vi "Select Measurement Listbox.vi"(6 "Cluster in":T3, 8 "error in (no error)":errorcluster, 9 "ThresholdLimits":refnum<vi>, 10 "Coords":T4, 11 "References in":T1) -> (0 "error out":errorcluster, 1 "Enable Disable button state":bool, 2 "Tick Marked?":bool, 3 "Cluster out":T3)   [LabVIEW 2019, in "ZenGage v3.0 UI.lvclass"]
doc: "This VI identifies selection of measurement in list and displays corresponding Lower Limit, Upper Limit, Lower Control Limit and Upper Control Limit values."
uses:
  ZenGage v3.0 UI.lvclass
  <vilib>/Utility/miscctls.llb/LVPositionTypeDef.ctl
  <vilib>/Utility/miscctls.llb/LVPoint32TypeDef.ctl
panel:
  out "References in":T1
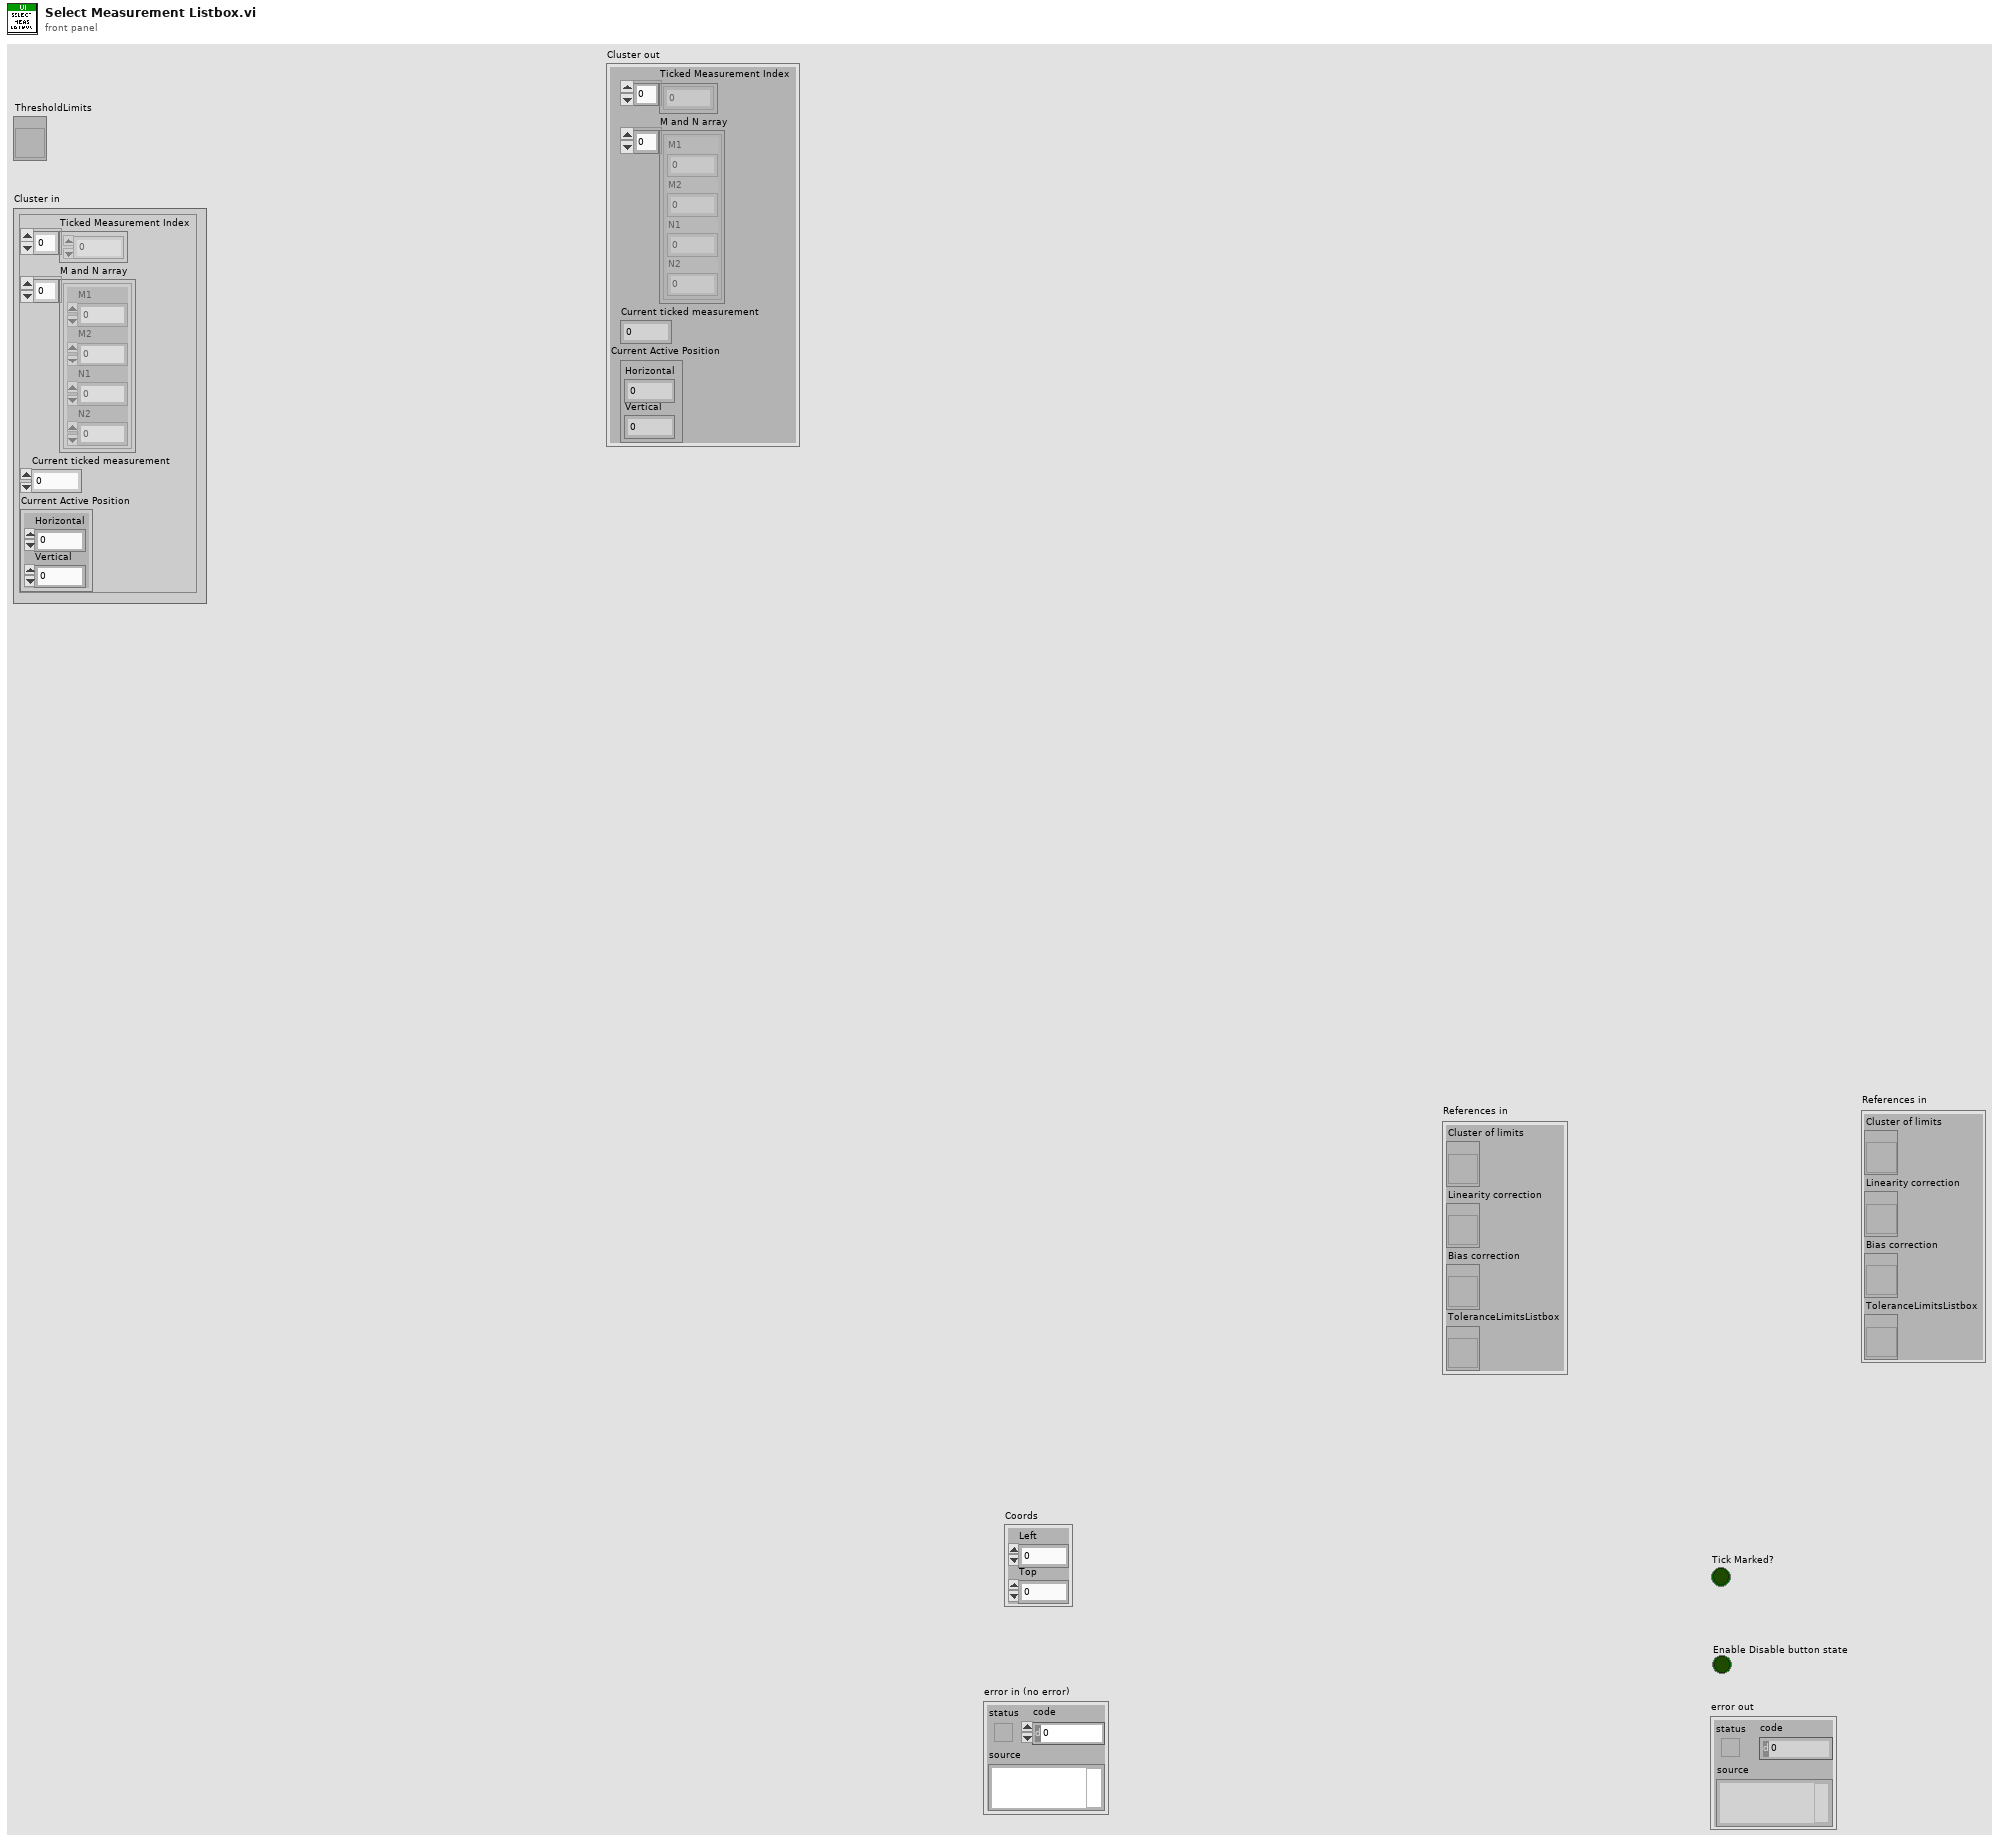
[diagram p1: front panel]
types:
  T1 = cluster{"Cluster of limits":refnum<vi>, "Linearity correction":refnum<vi>, "Bias correction":refnum<vi>, "ToleranceLimitsListbox":refnum<vi>}
  T2 = typedef "LVPoint32TypeDef.ctl" = cluster{"Horizontal":i32, "Vertical":i32}
  T3 = cluster{"Ticked Measurement Index":u32[], "M and N array":cluster{"M1":u64, "M2":u64, "N1":u64, "N2":u64}[], "Current ticked measurement":dbl, "Current Active Position":T2}
  T4 = typedef "LVPositionTypeDef.ctl" = cluster{"Left":i32, "Top":i32}
  T5 = cluster{"Lower Limit":dbl, "Upper Limit":dbl, "Lower Control Limit":dbl, "Upper Control Limit":dbl}
  T6 = enum8{"Enabled", "Disabled", "Disabled and Grayed Out"}
  T7 = cluster{"M1":u64, "M2":u64, "N1":u64, "N2":u64}[]
  T8 = typedef "LVRowAndColumnTypeDef.ctl" = cluster{"Row":i32, "Column":i32}
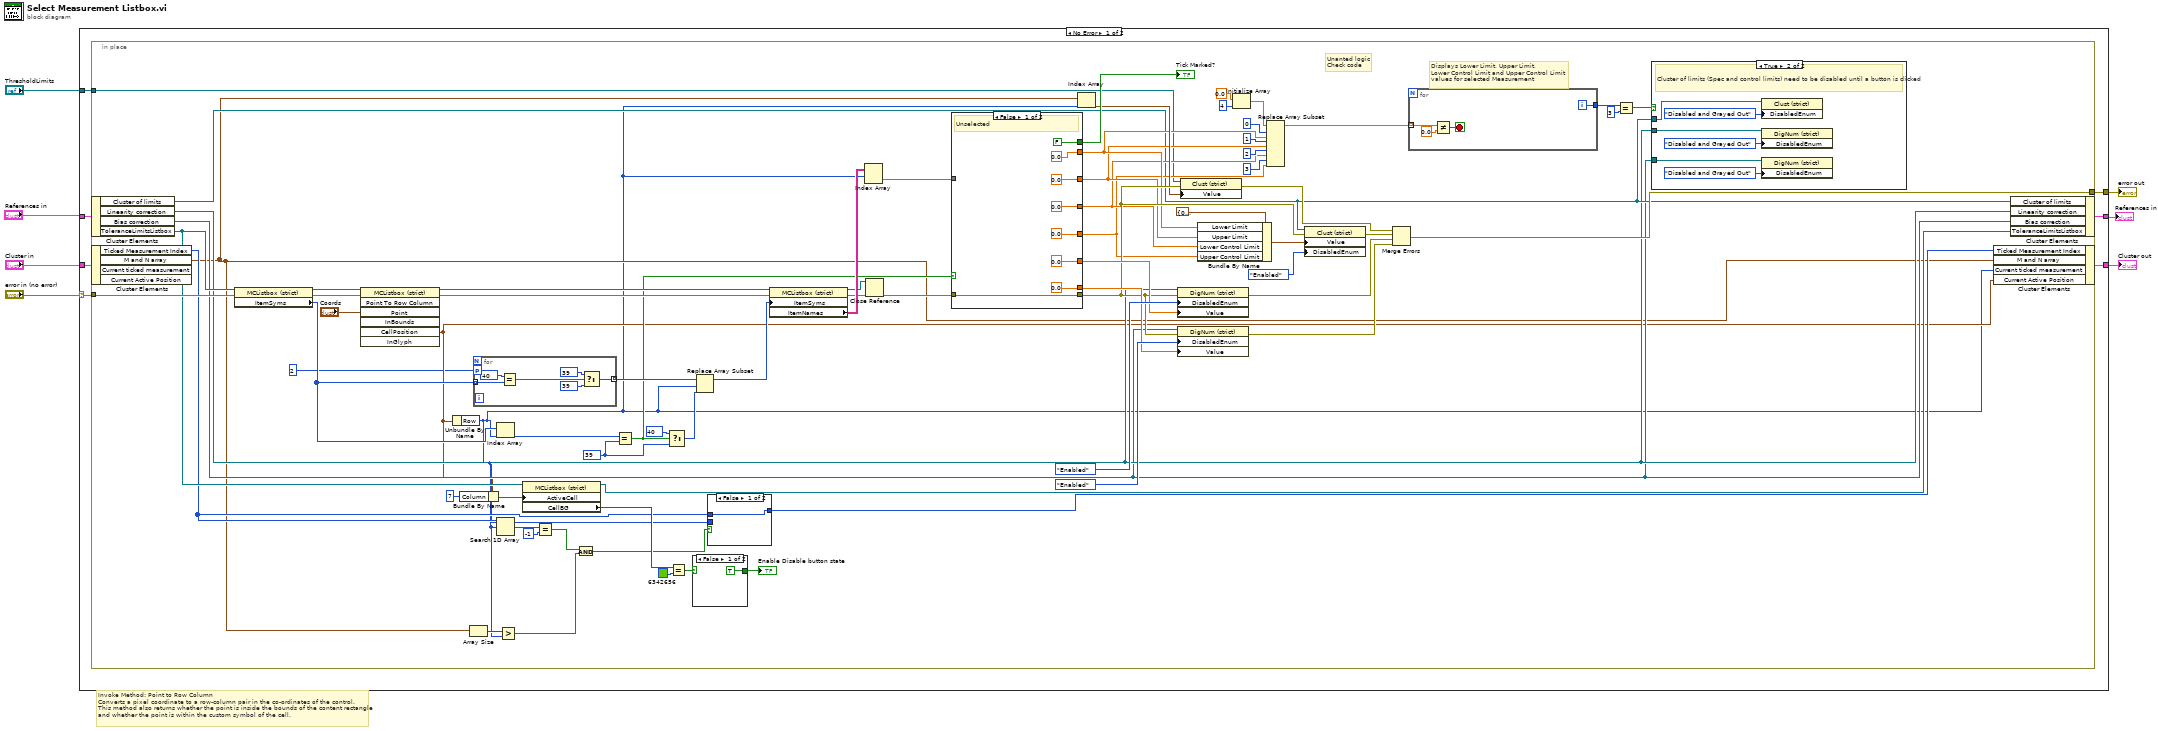
[diagram p0: block diagram]
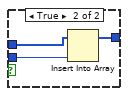
[diagram p2: hidden frame]
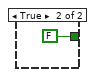
[diagram p3: hidden frame]
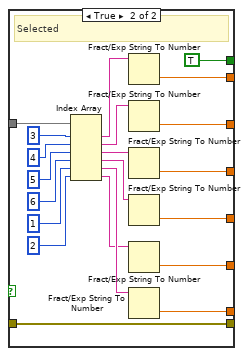
[diagram p5: hidden frame]
diagram:
  # "Invoke Method: Point to Row Column\nConverts a pixel coordinate to a row-column pair in the co-ordinates of the control.\nThis method also returns whether the point is inside the bounds of the content rectangle\nand whether the point is within the custom symbol of the cell."
  n1 = case shown="No Error" "error in (no error)" {
    selector: "error in (no error)" -> [w14 w141]
    tunnel: [w13 w141] -> w6
    tunnel: [w11 w140] -> w1
    tunnel: "References in" -> [w12 w140]
    tunnel: "ThresholdLimits" -> [w10 _]
    tunnel: "Cluster in" -> [w9 w139]
    tunnel: [w8 w139] -> w3
    frame No Error {
      n2 = in-place {
        in-place-border: w14 -> [w49]
        in-place-border: [w47] -> w13
        in-place-border: w10 -> [w25]
        w77 = 39
        # "Unanted logic\nCheck code"
        # "Displays Lower Limit, Upper Limit,\nLower Control Limit and Upper Control Limit\nvalues for selected Measurement"
        n3 = in-place-cluster #1(w12) -> ("Cluster of limits"=w29:refnum<vi>, "Linearity correction"=w28:refnum<vi>, "Bias correction"=w27:refnum<vi>, "ToleranceLimitsListbox"=w30:refnum<vi>)
        n4 = in-place-cluster #2(w9) -> ("Ticked Measurement Index"=w24:u32[], "M and N array"=w18:T7)  [unwired: 2 out]
        n5 = property on="Property Node" class="MCListbox (strict)"(reference=w30, error in=w49) -> (reference out=w85:refnum<vi>, error out=w86:errorcluster, "ItemSyms"=w75:i32[])
        n6 = invoke on="Invoke Node" class="MCListbox (strict)" method="Point To Row Column"(reference=w85, error in=w86, "Point"="Coords") -> (reference out=w84:refnum<vi>, error out=w83:errorcluster, "CellPosition"=w22:T8)  [unwired: 4 in, 4 out]
        n7 = Unbundle By Name(w22) -> ("Row"=w17:i32)
        n8 = Bundle By Name(cluster=w22, "Column"=7) -> (w50:T8)
        n9 = Array Size(array=w18) -> (size(s)=w19:i32)
        n10 = for {
          tunnel: w75 -> [w138] mode=indexing
          tunnel: [w134] -> w74 mode=indexing
          workers-P: 2 -> [_]
          n11 = Equal?(x=40, y=w138) -> (x = y?=w136:bool)
          n12 = Select(t=39, s=w136, f=39) -> (s? t:f=w134:i32)
        }
        n13 = Index Array "Index Array"(array=w75, index=w17) -> (element=w79:i32)
        n14 = Search 1D Array(1D array=w24, element=w17) -> (index of element=w37:i32)  [unwired: 1 in]
        n15 = Greater?(x=w19, y=w17) -> (0:w16:bool)
        n16 = property class="MCListbox (strict)"(reference=w30, "ActiveCell"=w50) -> (reference out=w26:refnum<vi>, "CellBG"=w54:u32)  [unwired: 1 in, 1 out]
        n17 = Equal?(x=w37, y=-1) -> (x = y?=w20:bool)
        n18 = And(x=w20, y=w16) -> (x .and. y?=w15:bool)
        n19 = Equal?(x=w79, y=w77) -> (x = y?=w73:bool)
        n20 = Select(t=40, s=w73, f=w77) -> (s? t:f=w78:i32)
        n21 = Equal?(x=w54, y=u32 6342656) -> (x = y?=w53:bool)
        n22 = case shown="False" w53 {
          tunnel: [TRUE FALSE] -> w52
          frame False {
          }
          frame True {
          }
        }
        "Enable Disable button state" <- w52
        n23 = Replace Array Subset "Replace Array Subset"(array=w74, new element=w78, index=w17) -> (w82:i32[])
        n24 = case shown="False" w15 {
          tunnel: [w88 w91] -> w23
          tunnel: w24 -> [w88 w90]
          tunnel: w17 -> [_ w89]
          frame False {
          }
          frame True {
            n25 = Insert Into Array(array=w90, new element=w89) -> (w91:u32[])  [unwired: 1 in]
          }
        }
        n26 = property on="Property Node" class="MCListbox (strict)"(reference=w84, error in=w83, "ItemSyms"=w82) -> (reference out=w70:refnum<vi>, error out=w72:errorcluster, "ItemNames"=w81:string[][])
        n27 = Index Array(array=w81, index (row)=w17) -> (element=w80:string[])  [unwired: 1 in]
        n28 = Close Reference(reference=w70, error in (no error)=w72) -> (error out=w71:errorcluster)
        n29 = case shown="False" w73 {
          tunnel: w80 -> [_ w132]
          tunnel: [0.0 w123] -> w35
          tunnel: [0.0 w122] -> w34
          tunnel: [0.0 w121] -> w33
          tunnel: [0.0 w120] -> w32
          tunnel: w71 -> [w107 w119]
          tunnel: [w107 w119] -> w40
          tunnel: [FALSE TRUE] -> w56
          tunnel: [0.0 w113] -> w42
          tunnel: [0.0 w112] -> w41
          frame False {
            # "Unselected"
          }
          frame True {
            # "Selected"
            n30 = Index Array(array=w132, index #1=3 ("index"), index #2=4 ("index"), index #3=5 ("index"), index #4=6 ("index"), index #5=1 ("index"), index #6=2 ("index")) -> (element #1=w127:string, element #2=w126:string, element #3=w125:string, element #4=w124:string, element #5=w115:string, element #6=w114:string)
            n31 = Fract/Exp String To Number(string=w127) -> (number=w123:dbl)  [unwired: 3 in, 1 out]
            n32 = Fract/Exp String To Number(string=w126) -> (number=w122:dbl)  [unwired: 3 in, 1 out]
            n33 = Fract/Exp String To Number(string=w125) -> (number=w121:dbl)  [unwired: 3 in, 1 out]
            n34 = Fract/Exp String To Number(string=w124) -> (number=w120:dbl)  [unwired: 3 in, 1 out]
            n35 = Fract/Exp String To Number(string=w114) -> (number=w112:dbl)  [unwired: 3 in, 1 out]
            n36 = Fract/Exp String To Number(string=w115) -> (number=w113:dbl)  [unwired: 3 in, 1 out]
          }
        }
        "Tick Marked?" <- w56
        n37 = Index Array(array=w18, index=w17) -> (element=w39:cluster{"M1":u64, "M2":u64, "N1":u64, "N2":u64})
        n38 = property class="DigNum (strict)"(reference=w28, error in=w40, "DisabledEnum"=T6."Enabled" ("Disabled"), "Value"=w41) -> (error out=w45:errorcluster)  [unwired: 1 out]
        n39 = property class="DigNum (strict)"(reference=w27, error in=w40, "DisabledEnum"=T6."Enabled" ("Disabled"), "Value"=w42) -> (error out=w43:errorcluster)  [unwired: 1 out]
        n40 = property class="Clust (strict)"(reference=w25, error in=w40, "Value"=w39) -> (error out=w38:errorcluster)  [unwired: 1 out]
        n41 = Bundle By Name(cluster=T5 {"Lower Limit"=0.0, "Upper Limit"=0.0, "Lower Control Limit"=0.0, "Upper Control Limit"=0.0} ("Value"), "Lower Limit"=w35, "Upper Limit"=w34, "Lower Control Limit"=w33, "Upper Control Limit"=w32) -> (w69:T5)
        n42 = Initialize Array(0.0, 4 ("dimension size")) -> (w66:dbl[])
        n43 = Replace Array Subset "Replace Array Subset"(array=w66, new element #1=w35, index #1=0 ("index"), new element #2=w34, index #2=1 ("index"), new element #3=w33, index #3=2 ("index"), new element #4=w32, index #4=3 ("index")) -> (w65:dbl[])
        n44 = property class="Clust (strict)"(reference=w29, error in=w40, "Value"=w69, "DisabledEnum"=T6."Enabled" ("Disabled")) -> (error out=w48:errorcluster)  [unwired: 1 out]
        n45 = Merge Errors(w38, w48, w45, w43) -> (w47:errorcluster)
        n46 = for {
          tunnel: w65 -> [w96] mode=indexing
          tunnel: [w97] -> w64
          i -> [w97]
          stop <- w94 stop-if-true
          n47 = Not Equal?(x=w96, y=0.0) -> (x != y?=w94:bool)
        }
        n48 = Equal?(x=w64, y=3) -> (x = y?=w62:bool)
        n49 = case shown="True" w62 {
          tunnel: w29 -> [_ w103]
          tunnel: w28 -> [_ w101]
          tunnel: w27 -> [_ w98]
          frame False {
          }
          frame True {
            # "Cluster of limits (Spec and control limits) need to be disabled until a button is clicked"
            n50 = property class="Clust (strict)"(reference=w103, "DisabledEnum"=T6."Disabled and Grayed Out" ("Disabled")) -> ()  [unwired: 1 in, 2 out]
            n51 = property class="DigNum (strict)"(reference=w101, "DisabledEnum"=T6."Disabled and Grayed Out" ("Disabled")) -> ()  [unwired: 1 in, 2 out]
            n52 = property class="DigNum (strict)"(reference=w98, "DisabledEnum"=T6."Disabled and Grayed Out" ("Disabled")) -> ()  [unwired: 1 in, 2 out]
          }
        }
        n53 = in-place-cluster #2("Ticked Measurement Index"=w23, "M and N array"=w18, "Current ticked measurement"=w17, "Current Active Position"=w22) -> (w8:T3)
        n54 = in-place-cluster #1("Cluster of limits"=w29, "Linearity correction"=w28, "Bias correction"=w27, "ToleranceLimitsListbox"=w26) -> (w11:T1)
      }
    }
    frame Error {
    }
  }
  "error out" <- w6
  "Cluster out" <- w3
  "References in" <- w1
